vi "Couter Read-Write.vi"(0 "File path":T1={"Wiker file"=path "E:/My Project/2018-2019/Under development/Minda Ind. Switch -ID 140-141/Project/data/Configuration Files/Station-1/Counter/handelbar/FeatureList-Winker.bin", "Horn file"=path "E:/My Project/2018-2019/Under development/Minda Ind. Switch -ID 140-141/Project/data/Configuration Files/Station-1/Counter/handelbar/FeatureList-Horn.bin", "Passing file"=path "E:/My Project/2018-2019/Under development/Minda Ind. Switch -ID 140-141/Project/data/Configuration Files/Station-1/Counter/handelbar/FeatureList-Passing.bin", "Dipper(Stepper) file"=path "E:/My Project/2018-2019/Under development/Minda Ind. Switch -ID 140-141/Project/data/Configuration Files/Station-1/Counter/handelbar/FeatureList-Dipper(Stepper).bin", "Light file"=path "E:/My Project/2018-2019/Under development/Minda Ind. Switch -ID 140-141/Project/data/Configuration Files/Station-1/Counter/handelbar/FeatureList-Light.bin", "Engine Start file"=path "E:/My Project/2018-2019/Under development/Minda Ind. Switch -ID 140-141/Project/data/Configuration Files/Station-1/Counter/handelbar/FeatureList-Engine Start.bin", "Hazard file"=path "E:/My Project/2018-2019/Under development/Minda Ind. Switch -ID 140-141/Project/data/Configuration Files/Station-1/Counter/handelbar/FeatureList-Hazard.bin"}, 5 "Data in":T2={"Set Counter"={"Set-Winker"=200, "Set-Horn"=300, "Set-Passing"=400, "Set-Dipper"=500, "Set-Light"=600, "Set-Enginestart"=700, "Set-Hazard"=800}, "Actual counter"={"Winker"=0, "Horn"=0, "Passing"=0, "Dipper"=0, "Light"=0, "Enginestart"=0, "Hazard"=0}}, 9 "Enum":enum16{"Read", "Write"}(ring)) -> (6 "Data out":T2, 15 "error out":errorcluster)   [LabVIEW 2015]
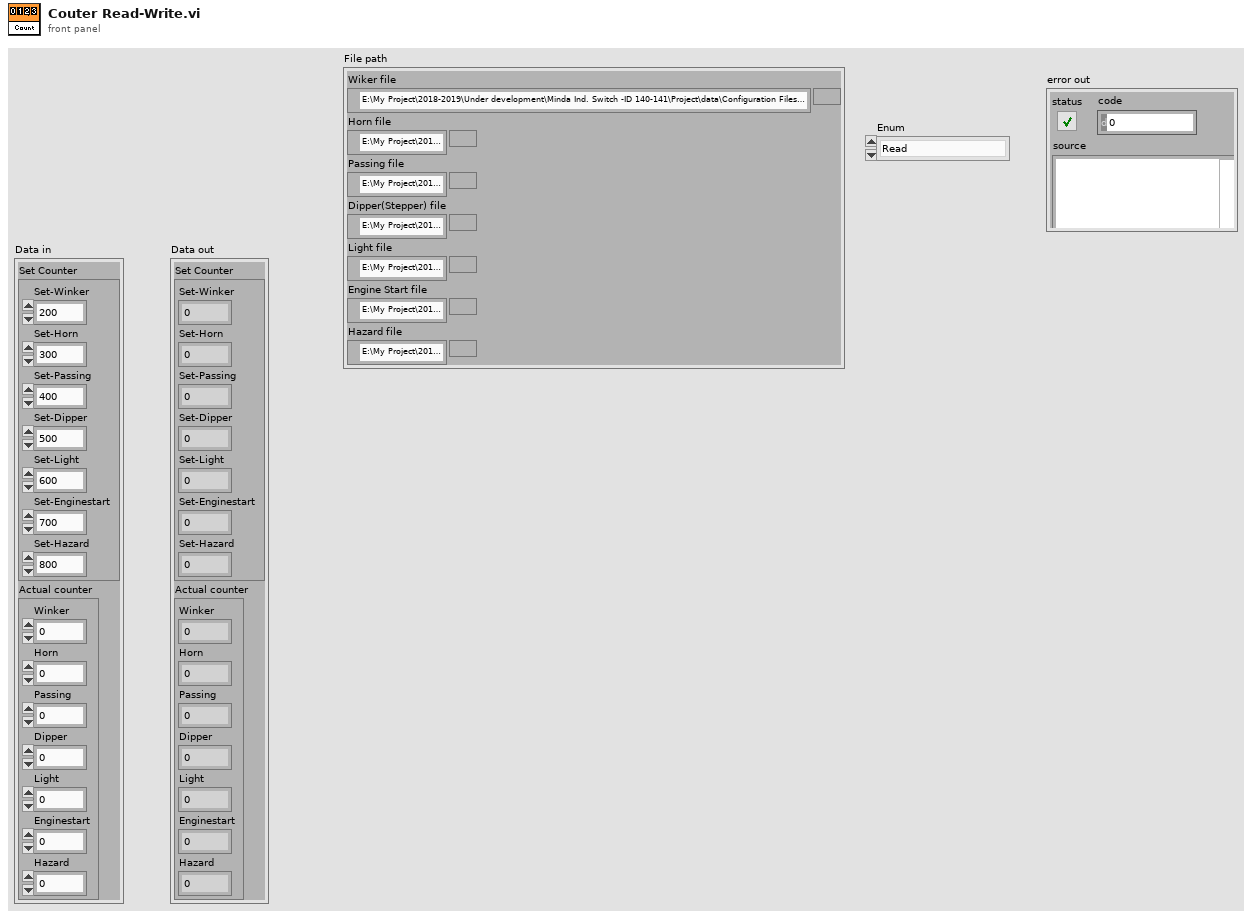
[diagram p1: front panel]
types:
  T1 = cluster{"Wiker file":path, "Horn file":path, "Passing file":path, "Dipper(Stepper) file":path, "Light file":path, "Engine Start file":path, "Hazard file":path}
  T2 = cluster{"Set Counter":cluster{"Set-Winker":i32, "Set-Horn":i32, "Set-Passing":i32, "Set-Dipper":i32, "Set-Light":i32, "Set-Enginestart":i32, "Set-Hazard":i32}, "Actual counter":cluster{"Winker":i32, "Horn":i32, "Passing":i32, "Dipper":i32, "Light":i32, "Enginestart":i32, "Hazard":i32}}
  T3 = cluster{"Winker":i32, "Horn":i32, "Passing":i32, "Dipper":i32, "Light":i32, "Enginestart":i32, "Hazard":i32}
  T4 = cluster{"Set-Winker":i32, "Set-Horn":i32, "Set-Passing":i32, "Set-Dipper":i32, "Set-Light":i32, "Set-Enginestart":i32, "Set-Hazard":i32}
  T5 = cluster{"Set-Enginestart":i32, "Enginestart":i32}
  T6 = enum16{"open", "replace", "create", "open or create", "replace or create", "replace or create with confirmation"}
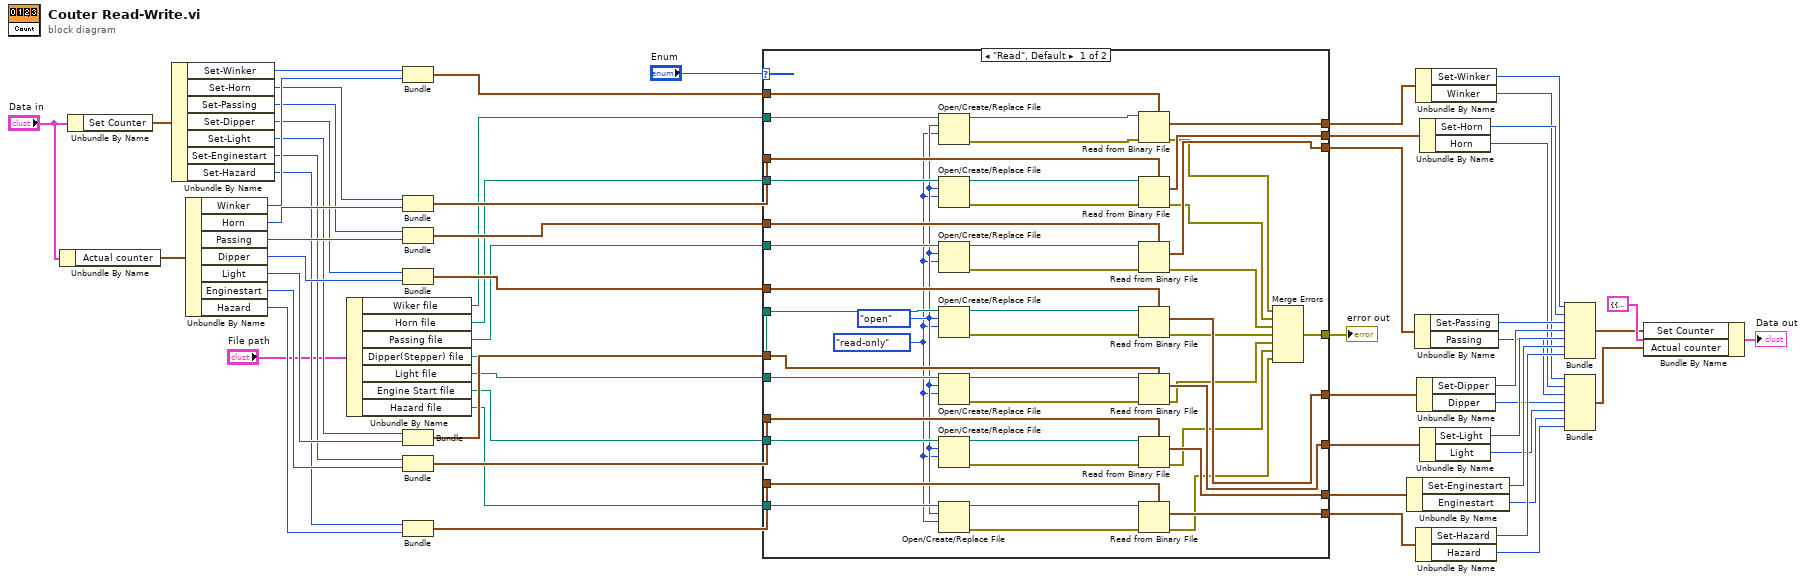
[diagram p0: block diagram]
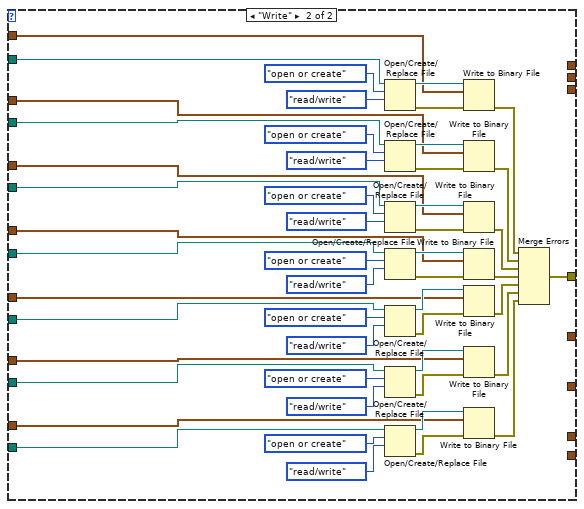
[diagram p2: hidden frame]
diagram:
  n1 = Unbundle By Name("Data in") -> ("Actual counter"=w55:T3)
  n2 = Unbundle By Name("Data in") -> ("Set Counter"=w57:T4)
  n3 = Unbundle By Name(w57) -> ("Set-Winker"=w54:i32, "Set-Horn"=w52:i32, "Set-Passing"=w50:i32, "Set-Dipper"=w48:i32, "Set-Light"=w46:i32, "Set-Enginestart"=w44:i32, "Set-Hazard"=w42:i32)
  n4 = Unbundle By Name(w55) -> ("Winker"=w53:i32, "Horn"=w51:i32, "Passing"=w49:i32, "Dipper"=w47:i32, "Light"=w45:i32, "Enginestart"=w43:i32, "Hazard"=w41:i32)
  n5 = Unbundle By Name("File path") -> ("Wiker file"=w9:path, "Horn file"=w8:path, "Passing file"=w7:path, "Dipper(Stepper) file"=w6:path, "Light file"=w5:path, "Engine Start file"=w4:path, "Hazard file"=w3:path)
  n6 = Bundle("Set-Winker"=w54, "Winker"=w53) -> (w40:cluster{"Set-Winker":i32, "Winker":i32})  [unwired: 1 in]
  n7 = Bundle("Set-Horn"=w52, "Horn"=w51) -> (w39:cluster{"Set-Horn":i32, "Horn":i32})  [unwired: 1 in]
  n8 = Bundle("Set-Passing"=w50, "Passing"=w49) -> (w38:cluster{"Set-Passing":i32, "Passing":i32})  [unwired: 1 in]
  n9 = Bundle("Set-Dipper"=w48, "Dipper"=w47) -> (w37:cluster{"Set-Dipper":i32, "Dipper":i32})  [unwired: 1 in]
  n10 = Bundle("Set-Light"=w46, "Light"=w45) -> (w36:cluster{"Set-Light":i32, "Light":i32})  [unwired: 1 in]
  n11 = Bundle("Set-Enginestart"=w44, "Enginestart"=w43) -> (w35:T5)  [unwired: 1 in]
  n12 = Bundle("Set-Hazard"=w42, "Hazard"=w41) -> (w34:cluster{"Set-Hazard":i32, "Hazard":i32})  [unwired: 1 in]
  n13 = case shown="\"Read\", Default" "Enum" {
    tunnel: w9 -> [w104 w150]
    tunnel: [w69 w105] -> w58
    tunnel: w8 -> [w89 w129]
    tunnel: w7 -> [w88 w128]
    tunnel: w6 -> [w87 w127]
    tunnel: w5 -> [w86 w126]
    tunnel: w4 -> [w85 w125]
    tunnel: w3 -> [w84 w120]
    tunnel: w40 -> [w83 w114]
    tunnel: w39 -> [w82 w113]
    tunnel: w38 -> [w81 w119]
    tunnel: w37 -> [w80 w118]
    tunnel: w36 -> [w79 w117]
    tunnel: w35 -> [w78 w116]
    tunnel: w34 -> [w77 w115]
    tunnel: [w76 _] -> w33
    tunnel: [w75 _] -> w32
    tunnel: [w74 _] -> w31
    tunnel: [w73 _] -> w30
    tunnel: [w72 _] -> w29
    tunnel: [w71 _] -> w28
    tunnel: [w70 _] -> w27
    frame "Read", Default {
      w67 = enum16{"read/write", "read-only", "write-only"}."read-only" ("access (0:read/write)")
      w68 = T6."open" ("operation (0:open)")
      n14 = Open/Create/Replace File(file path (use dialog)=w104, operation (0:open)=w68, access (0:read/write)=w67) -> (refnum out=w103:refnum<file>, error out=w102:errorcluster)  [unwired: 3 in, 1 out]
      n15 = Open/Create/Replace File(file path (use dialog)=w89, operation (0:open)=w68, access (0:read/write)=w67) -> (refnum out=w100:refnum<file>, error out=w101:errorcluster)  [unwired: 3 in, 1 out]
      n16 = Open/Create/Replace File(file path (use dialog)=w88, operation (0:open)=w68, access (0:read/write)=w67) -> (refnum out=w99:refnum<file>, error out=w98:errorcluster)  [unwired: 3 in, 1 out]
      n17 = Open/Create/Replace File(file path (use dialog)=w87, operation (0:open)=w68, access (0:read/write)=w67) -> (refnum out=w96:refnum<file>, error out=w97:errorcluster)  [unwired: 3 in, 1 out]
      n18 = Open/Create/Replace File(file path (use dialog)=w86, operation (0:open)=w68, access (0:read/write)=w67) -> (refnum out=w95:refnum<file>, error out=w94:errorcluster)  [unwired: 3 in, 1 out]
      n19 = Open/Create/Replace File(file path (use dialog)=w85, operation (0:open)=w68, access (0:read/write)=w67) -> (refnum out=w92:refnum<file>, error out=w93:errorcluster)  [unwired: 3 in, 1 out]
      n20 = Open/Create/Replace File(file path (use dialog)=w84, operation (0:open)=w68, access (0:read/write)=w67) -> (refnum out=w91:refnum<file>, error out=w90:errorcluster)  [unwired: 3 in, 1 out]
      n21 = Read from Binary File(5:w83, 8:w102, 11:w103) -> (0:w64:errorcluster, 2:w76:cluster{"Set-Winker":i32, "Winker":i32})  [unwired: 3 in, 2 out]
      n22 = Read from Binary File(5:w82, 8:w101, 11:w100) -> (0:w65:errorcluster, 2:w75:cluster{"Set-Horn":i32, "Horn":i32})  [unwired: 3 in, 2 out]
      n23 = Read from Binary File(5:w81, 8:w98, 11:w99) -> (0:w66:errorcluster, 2:w74:cluster{"Set-Passing":i32, "Passing":i32})  [unwired: 3 in, 2 out]
      n24 = Read from Binary File(5:w80, 8:w97, 11:w96) -> (0:w63:errorcluster, 2:w73:cluster{"Set-Dipper":i32, "Dipper":i32})  [unwired: 3 in, 2 out]
      n25 = Read from Binary File(5:w79, 8:w94, 11:w95) -> (0:w62:errorcluster, 2:w72:cluster{"Set-Light":i32, "Light":i32})  [unwired: 3 in, 2 out]
      n26 = Read from Binary File(5:w78, 8:w93, 11:w92) -> (0:w61:errorcluster, 2:w71:T5)  [unwired: 3 in, 2 out]
      n27 = Read from Binary File(5:w77, 8:w90, 11:w91) -> (0:w60:errorcluster, 2:w70:cluster{"Set-Hazard":i32, "Hazard":i32})  [unwired: 3 in, 2 out]
      n28 = Merge Errors(w64, w65, w66, w63, w62, w61, w60) -> (w69:errorcluster)
    }
    frame "Write" {
      n29 = Open/Create/Replace File(file path (use dialog)=w150, operation (0:open)=T6."open or create", access (0:read/write)=enum16{"read/write", "read-only", "write-only"}."read/write") -> (refnum out=w152:refnum<file>, error out=w151:errorcluster)  [unwired: 3 in, 1 out]
      n30 = Open/Create/Replace File(file path (use dialog)=w129, operation (0:open)=T6."open or create", access (0:read/write)=enum16{"read/write", "read-only", "write-only"}."read/write") -> (refnum out=w148:refnum<file>, error out=w149:errorcluster)  [unwired: 3 in, 1 out]
      n31 = Open/Create/Replace File(file path (use dialog)=w128, operation (0:open)=T6."open or create", access (0:read/write)=enum16{"read/write", "read-only", "write-only"}."read/write") -> (refnum out=w143:refnum<file>, error out=w142:errorcluster)  [unwired: 3 in, 1 out]
      n32 = Open/Create/Replace File(file path (use dialog)=w127, operation (0:open)=T6."open or create", access (0:read/write)=enum16{"read/write", "read-only", "write-only"}."read/write") -> (refnum out=w140:refnum<file>, error out=w141:errorcluster)  [unwired: 3 in, 1 out]
      n33 = Open/Create/Replace File(file path (use dialog)=w126, operation (0:open)=T6."open or create", access (0:read/write)=enum16{"read/write", "read-only", "write-only"}."read/write") -> (refnum out=w135:refnum<file>, error out=w134:errorcluster)  [unwired: 3 in, 1 out]
      n34 = Open/Create/Replace File(file path (use dialog)=w125, operation (0:open)=T6."open or create", access (0:read/write)=enum16{"read/write", "read-only", "write-only"}."read/write") -> (refnum out=w132:refnum<file>, error out=w133:errorcluster)  [unwired: 3 in, 1 out]
      n35 = Open/Create/Replace File(file path (use dialog)=w120, operation (0:open)=T6."open or create", access (0:read/write)=enum16{"read/write", "read-only", "write-only"}."read/write") -> (refnum out=w122:refnum<file>, error out=w121:errorcluster)  [unwired: 3 in, 1 out]
      n36 = Write to Binary File(file (use dialog)=w152, data=w114, error in=w151) -> (error out=w112:errorcluster)  [unwired: 3 in, 2 out]
      n37 = Write to Binary File(file (use dialog)=w148, data=w113, error in=w149) -> (error out=w111:errorcluster)  [unwired: 3 in, 2 out]
      n38 = Write to Binary File(file (use dialog)=w143, data=w119, error in=w142) -> (error out=w110:errorcluster)  [unwired: 3 in, 2 out]
      n39 = Write to Binary File(file (use dialog)=w140, data=w118, error in=w141) -> (error out=w109:errorcluster)  [unwired: 3 in, 2 out]
      n40 = Write to Binary File(file (use dialog)=w135, data=w117, error in=w134) -> (error out=w108:errorcluster)  [unwired: 3 in, 2 out]
      n41 = Write to Binary File(file (use dialog)=w132, data=w116, error in=w133) -> (error out=w107:errorcluster)  [unwired: 3 in, 2 out]
      n42 = Write to Binary File(file (use dialog)=w122, data=w115, error in=w121) -> (error out=w106:errorcluster)  [unwired: 3 in, 2 out]
      n43 = Merge Errors(w112, w111, w110, w109, w108, w107, w106) -> (w105:errorcluster)
    }
  }
  "error out" <- w58
  n44 = Unbundle By Name(w28) -> ("Set-Enginestart"=w21:i32, "Enginestart"=w14:i32)
  n45 = Unbundle By Name(w31) -> ("Set-Passing"=w24:i32, "Passing"=w17:i32)
  n46 = Unbundle By Name(w33) -> ("Set-Winker"=w26:i32, "Winker"=w19:i32)
  n47 = Unbundle By Name(w27) -> ("Set-Hazard"=w20:i32, "Hazard"=w13:i32)
  n48 = Unbundle By Name(w30) -> ("Set-Dipper"=w23:i32, "Dipper"=w16:i32)
  n49 = Unbundle By Name(w32) -> ("Set-Horn"=w25:i32, "Horn"=w18:i32)
  n50 = Unbundle By Name(w29) -> ("Set-Light"=w22:i32, "Light"=w15:i32)
  n51 = Bundle("Set-Winker"=w26, "Set-Horn"=w25, "Set-Passing"=w24, "Set-Dipper"=w23, "Set-Light"=w22, "Set-Enginestart"=w21, "Set-Hazard"=w20) -> (w2:T4)  [unwired: 1 in]
  n52 = Bundle("Winker"=w19, "Horn"=w18, "Passing"=w17, "Dipper"=w16, "Light"=w15, "Enginestart"=w14, "Hazard"=w13) -> (w1:T3)  [unwired: 1 in]
  n53 = Bundle By Name(cluster=T2 {"Set Counter"={"Set-Winker"=0, "Set-Horn"=0, "Set-Passing"=0, "Set-Dipper"=0, "Set-Light"=0, "Set-Enginestart"=0, "Set-Hazard"=0}, "Actual counter"={"Winker"=0, "Horn"=0, "Passing"=0, "Dipper"=0, "Light"=0, "Enginestart"=0, "Hazard"=0}} ("Data out 2"), "Set Counter"=w2, "Actual counter"=w1) -> (→"Data out":T2)
